vi "Set Max ROI Overlay.vi"(8 "error in (no error)":errorcluster, 10 "Max Gauge ROI":T2, 11 "Image in":T1) -> (0 "error out":errorcluster, 3 "Image out":T1)   [LabVIEW 2011, in "Meter Detection Custom Device.lvlib"]
uses:
  Meter Detection Custom Device.lvlib
  <vilib>/vision/Image Controls.llb/IMAQ Image.ctl
  Meter Detection Global Variable.vi
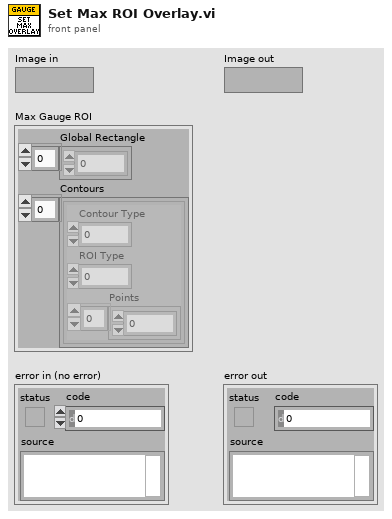
[diagram p1: front panel]
types:
  T1 = typedef "IMAQ Image.ctl" = refnum<image>
  T2 = cluster{"Global Rectangle":i32[], "Contours":cluster{"Contour Type":u32, "ROI Type":u32, "Points":i32[]}[]}
  T3 = cluster{"Desired Font (Application)":enum16{"User-specified Font", "Application Font", "System Font", "Dialog Font"}, "[User-specified Font]":cluster{"Font Name":string, "Size":i16, "Strikeout?":bool, "Italic?":bool, "Underline?":bool, "Outline?":bool, "Shadow?":bool, "Bold?":bool, "Rotation Angle":dbl}, "Horizontal Alignment":i16, "Vertical Alignment":i16}
  T4 = typedef "IMAQ Line" = cluster{"Start X":i32, "Start Y":i32, "End X":i32, "End Y":i32}
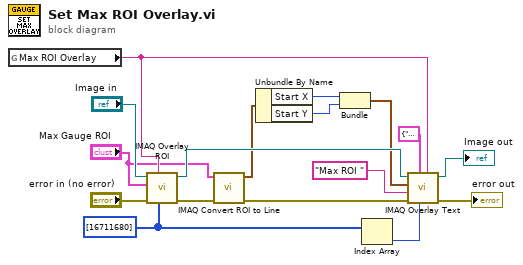
[diagram p0: block diagram]
diagram:
  w10 = u32[] [16711680] ("Colors (Green)")
  n1 = global read "Meter Detection Global Variable.vi" "Max ROI Overlay"() -> (w15:string)
  n2 = call "IMAQ Overlay ROI"("Colors (Green)"=w10, "Group"=w15, "error in (no error)"="error in (no error)", "ROI Descriptor"="Max Gauge ROI", "Image"="Image in") -> ("error out"=w8:errorcluster, "Image Out"=w12:T1)  [unwired: 5 in]
  n3 = call "IMAQ Convert ROI to Line"("error in (no error)"=w8, "ROI Descriptor"="Max Gauge ROI") -> ("error out"=w7:errorcluster, "Line"=w5:T4)  [unwired: 7 in]
  n4 = Unbundle By Name(w5) -> ("Start X"=w4:i32, "Start Y"=w3:i32)
  n5 = Bundle("Start X"=w4, "Start Y"=w3) -> (w2:cluster{"Start X":i32, "Start Y":i32})  [unwired: 1 in]
  n6 = Index Array(array=w10) -> (element=w9:u32)  [unwired: 1 in]
  n7 = call "IMAQ Overlay Text"("Group"=w15, "Text Color (black)"=w9, "Font, Size & Style"=T3 {"Desired Font (Application)"=enum."Application Font", "[User-specified Font]"={"Font Name"="", "Size"=12, "Strikeout?"=FALSE, "Italic?"=FALSE, "Underline?"=FALSE, "Outline?"=FALSE, "Shadow?"=FALSE, "Bold?"=FALSE, "Rotation Angle"=0.0}, "Horizontal Alignment"=1, "Vertical Alignment"=0}, "error in (no error)"=w7, "String"="Max ROI ", "Origin"=w2, "Image"=w12) -> ("error out"=→"error out":errorcluster, "Image Out"=→"Image out":T1)  [unwired: 3 in]
